vi "Add Parameter (Double) and Default Assignment.vi"(6 "Default Assignment":string, 7 "Evaluation Method (ByReference)":i32(ring)=1 items=["ByValue", "ByReference"], 8 "error in (no error)":errorcluster, 9 "Value":dbl, 10 "Identifier":string, 11 "Sequence Ref in":refnum<k24>) -> (0 "error out":errorcluster, 3 "Sequence Ref out":refnum<k24>)   [LabVIEW 2013, in "Simple Sequence Tools - Editor.lvlib"]
uses:
  NationalInstruments.VeriStand.RealTimeSequenceDefinitionApi
  NationalInstruments.VeriStand.DataTypes
  Simple Sequence Tools - Editor.lvlib
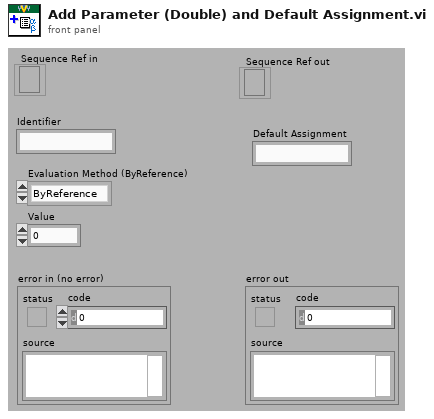
[diagram p1: front panel]
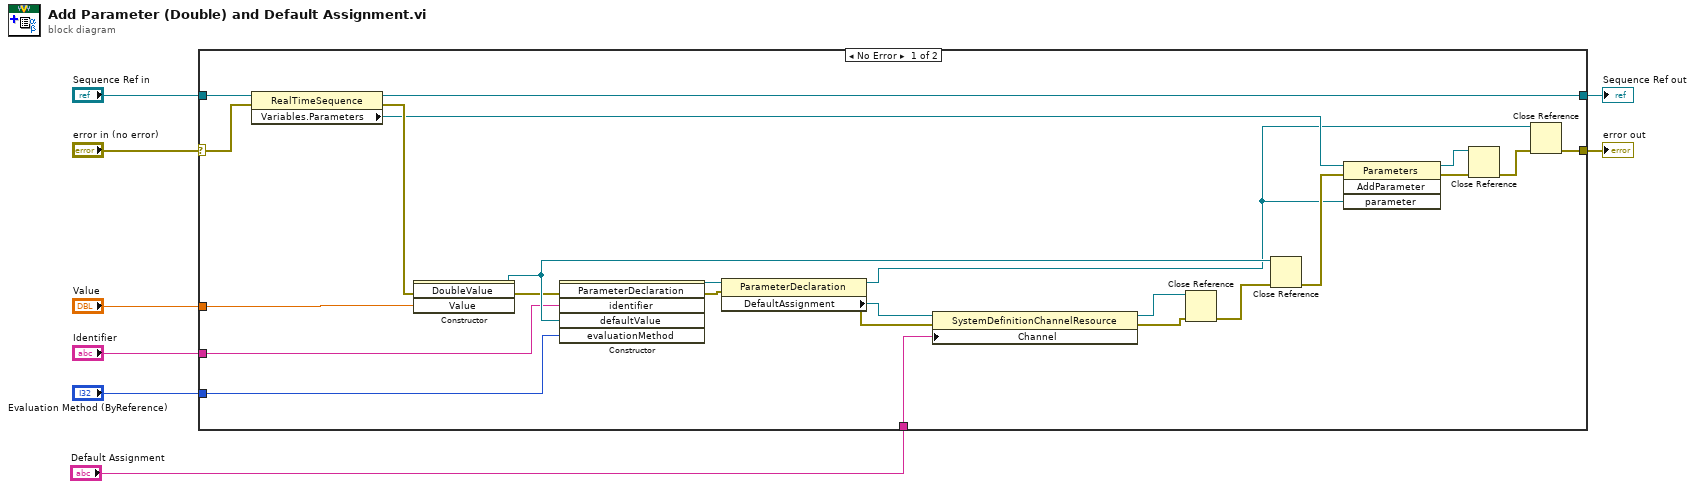
[diagram p0: block diagram]
diagram:
  n1 = case shown="No Error" "error in (no error)" {
    selector: "error in (no error)" -> [w18 w33]
    tunnel: "Value" -> [w29 _]
    tunnel: "Identifier" -> [w26 _]
    tunnel: "Evaluation Method (ByReference)" -> [w25 _]
    tunnel: "Sequence Ref in" -> [w24 w34]
    tunnel: [w23 w34] -> w4
    tunnel: [w20 w33] -> w3
    tunnel: "Default Assignment" -> [w13 _]
    frame No Error {
      n2 = property class="RealTimeSequence"(reference=w24, error in=w18) -> (reference out=w23:refnum<k24>, error out=w28:errorcluster, "Variables.Parameters"=w27:refnum<k24>)
      n3 = constructor class="DoubleValue"(error in=w28, "Value"=w29) -> (reference out=w31:refnum<k24>, error out=w30:errorcluster)  [unwired: 2 in, 2 out]
      n4 = constructor class="ParameterDeclaration"(error in=w30, "identifier"=w26, "defaultValue"=w31, "evaluationMethod"=w25) -> (reference out=w17:refnum<k24>, error out=w16:errorcluster)  [unwired: 2 in, 4 out]
      n5 = property class="ParameterDeclaration"(reference=w17, error in=w16) -> (reference out=w12:refnum<k24>, error out=w14:errorcluster, "DefaultAssignment"=w15:refnum<k24>)
      n6 = property class="SystemDefinitionChannelResource"(reference=w15, error in=w14, "Channel"=w13) -> (reference out=w10:refnum<k24>, error out=w11:errorcluster)
      n7 = Close Reference(reference=w10, error in (no error)=w11) -> (error out=w9:errorcluster)
      n8 = Close Reference(reference=w31, error in (no error)=w9) -> (error out=w32:errorcluster)
      n9 = invoke class="Parameters" method="AddParameter"(reference=w27, error in=w32, "parameter"=w12) -> (reference out=w19:refnum<k24>, error out=w22:errorcluster)  [unwired: 1 in, 2 out]
      n10 = Close Reference(reference=w19, error in (no error)=w22) -> (error out=w21:errorcluster)
      n11 = Close Reference(reference=w12, error in (no error)=w21) -> (error out=w20:errorcluster)
    }
    frame Error {
    }
  }
  "Sequence Ref out" <- w4
  "error out" <- w3
